vi "Prefilter.Low Pass.vi"(8 "error in (no error)":errorcluster, 9 "Low Pass Cutoff (Hz)":dbl, 10 "signal in":waveform(dbl)[](array[waveform]), 11 "DSP in":refnum<class "DSP.lvclass">) -> (0 "error out":errorcluster, 2 "signa out":waveform(dbl)[](array[waveform]), 3 "DSP out":refnum<class "DSP.lvclass">)   [LabVIEW 2019, in "DSP.lvclass"]
uses:
  DSP.lvclass
  DSP.lvclass/DSP.ctl
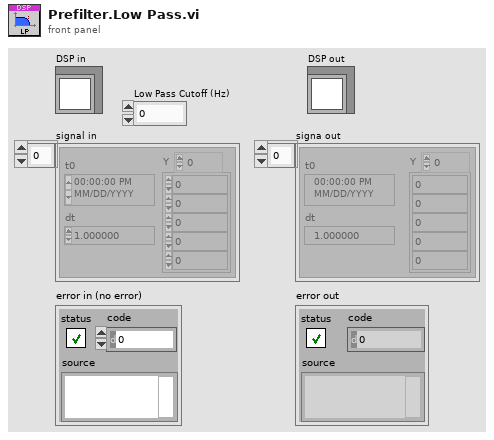
[diagram p1: front panel]
types:
  T1 = cluster{"filter structure":enum32{"IIR 2nd Order", "IIR 4th Order"}, "Reverse Coefficients":dbl[], "Forward Coefficients":dbl[]}[]
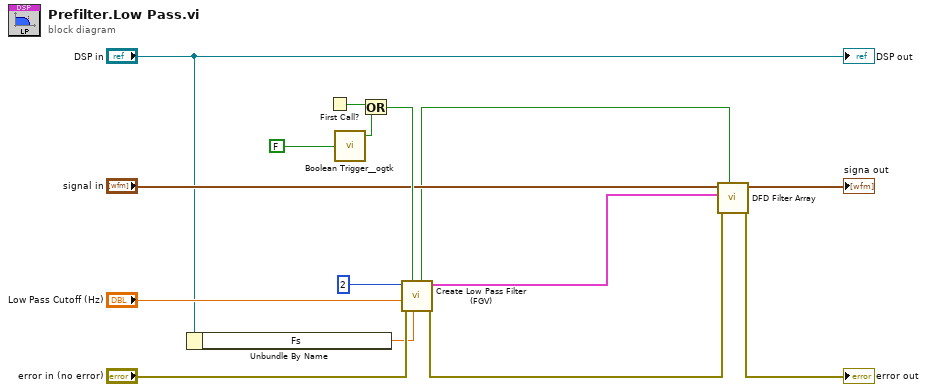
[diagram p0: block diagram]
diagram:
  n1 = Unbundle By Name("DSP in") -> ("Fs"=w3:dbl)
  n2 = First Call?() -> (First Call?: T/F=w13:bool)
  n3 = call <userlib>:"Boolean Trigger__ogtk.vi"("Boolean Input"=FALSE) -> ("Rising Edge"=w12:bool)  [unwired: 1 in, 1 out]
  n4 = Or(x=w13, y=w12) -> (x .or. y?=w11:bool)
  n5 = call "Create Low Pass Filter (FGV).vi"("fs (Hz)"=w3, "init [F]"=w11, "error in (no error)"="error in (no error)", "Low Pass Cutoff (Hz)"="Low Pass Cutoff (Hz)", "order"=2) -> ("error out"=w7:errorcluster, "IIR Filters"=w1:T1, "init out"=w6:bool)  [unwired: 4 in]
  n6 = call "DFD Filter Array.vi"("init (F)"=w6, "error in (no error)"=w7, "IIR Filters"=w1, "signal in"="signal in") -> ("error out"=→"error out":errorcluster, "signal out"=→"signa out":waveform(dbl)[])  [unwired: 6 in]
  "DSP out" <- "DSP in"
